vi "init.vi"(8 "error in":errorcluster, 10 "TBM module configuration in":refnum<class "TBM module configuration.lvclass">, 11 "Increment runtime in":refnum<class "Increment runtime.lvclass">) -> (0 "error out":errorcluster, 1 "data allocations":T1, 2 "execution settings":T4, 3 "Increment runtime out":refnum<class "Increment runtime.lvclass">)   [LabVIEW 2015, in "Increment runtime.lvclass"]
doc: "Provides an interface for initializing a module at runtime. While this interface performs no operations, a child should provide an override which may open any necessary references or sessions, allocate necessary memory, and perform any final configuration validataion before providing the full configuration <b>execution data</b> to the calling process."
uses:
  Increment runtime.lvclass
  <vilib>/NI/Tag Bus Module Framework/module configuration/TBM module configuration.lvclass
  <vilib>/NI/Tag Bus Module Framework/runtime/execution settings.ctl
  <vilib>/NI/Tag Bus Module Framework/channel/data tables.ctl
  <vilib>/NI/Tag Bus/dictionary/data dictionary.lvclass
  <vilib>/NI/Tag Bus/dictionary table pair.ctl
  <vilib>/NI/Tag Bus/table/data table.ctl
  configuration/Increment configuration.lvclass
  configuration/Increment configuration.lvclass/Increment configuration.ctl
  Runtime_Mapping.ctl
  <vilib>/NI/Tag Bus/tag/tag descriptor.lvclass/tag descriptor.ctl
  Increment runtime.lvclass/Increment runtime.ctl
  configuration/Read Lines.vi
  <vilib>/NI/Tag Bus/tag/read tag name.vi
  <vilib>/NI/Tag Bus/tag/read data type.vi
  <vilib>/NI/Tag Bus/dictionary/locate tag.vi
  <vilib>/NI/Tag Bus Module Framework/channel/TBM channel.lvclass
  <vilib>/NI/Tag Bus Module Framework/runtime/TBM module execution interface.lvclass
  <vilib>/NI/Tag Bus/tag bus.lvlib
  <vilib>/NI/Tag Bus/table/data table.lvlib
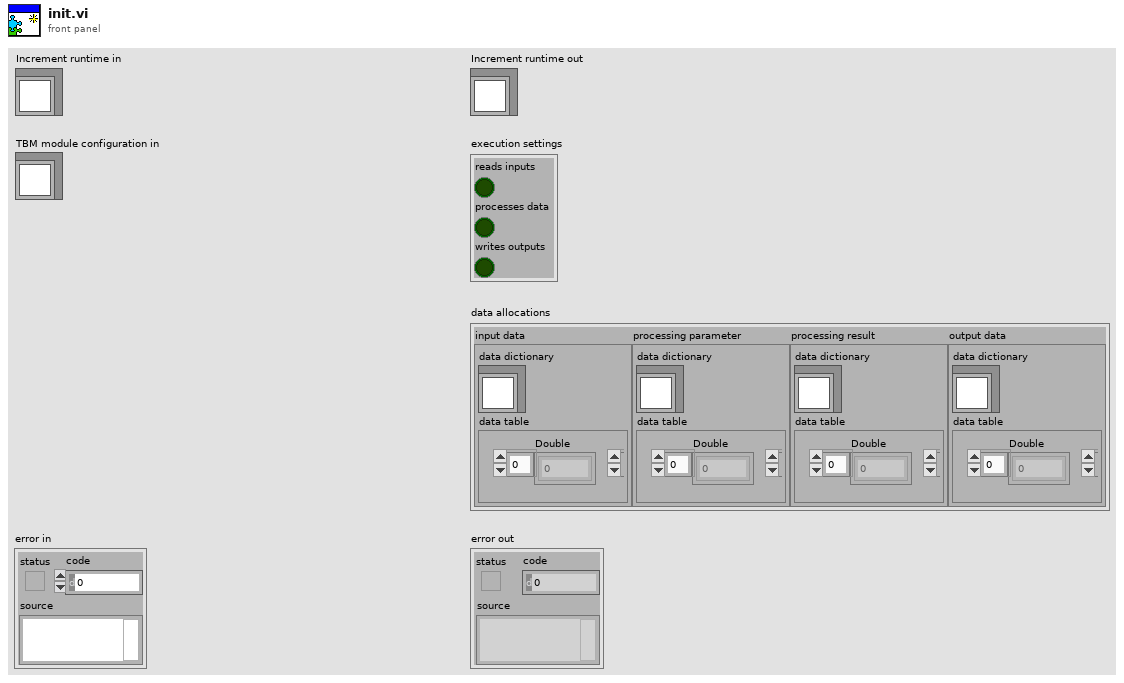
[diagram p1: front panel]
types:
  T1 = typedef "TBM channel.lvclass/data tables.ctl" = cluster{"input data":T2, "processing parameter":T2, "processing result":T2, "output data":T2}
  T2 = typedef "tag bus.lvlib/dictionary table pair.ctl" = cluster{"data dictionary":refnum<class "data dictionary.lvclass">, "data table":T3}
  T3 = typedef "tag bus.lvlib/data table.lvlib/data table.ctl" = cluster{"Double":dbl[], "Single":sgl[], "I64":i64[], "I32":i32[], "I16":i16[], "I8":i8[], "U64":u64[], "U32":u32[], "U16":u16[], "U8":u8[], "Boolean":bool[], "String":string[], "Array of Double":cluster{"DBL Array":dbl[]}[], "Array of Single":cluster{"SGL Array":sgl[]}[], "Array of I64":cluster{"I64 Array":i64[]}[], "Array of I32":cluster{"I32 Array":i32[]}[], "Array of I16":cluster{"I16 Array":i16[]}[], "Array of I8":cluster{"I8 Array":i8[]}[], "Array of U64":cluster{"U64 Array":u64[]}[], "Array of U32":cluster{"U32 Array":u32[]}[], "Array of U16":cluster{"U16 Array":u16[]}[], "Array of U8":cluster{"U8 Array":u8[]}[], "Array of Boolean":cluster{"Boolean Array":bool[]}[], "Array of String":cluster{"String Array":string[]}[]}
  T4 = typedef "TBM module execution interface.lvclass/execution settings.ctl" = cluster{"reads inputs":bool, "processes data":bool, "writes outputs":bool}
  T5 = typedef "Increment runtime.lvclass/Runtime_Mapping.ctl" = cluster{"In Index":i32, "Out Index":i32}
  T6 = typedef "Increment configuration.lvclass/Line.ctl" = cluster{"Name":string, "channel in":refnum<class "TBM channel.lvclass">, "channel out":refnum<class "TBM channel.lvclass">}
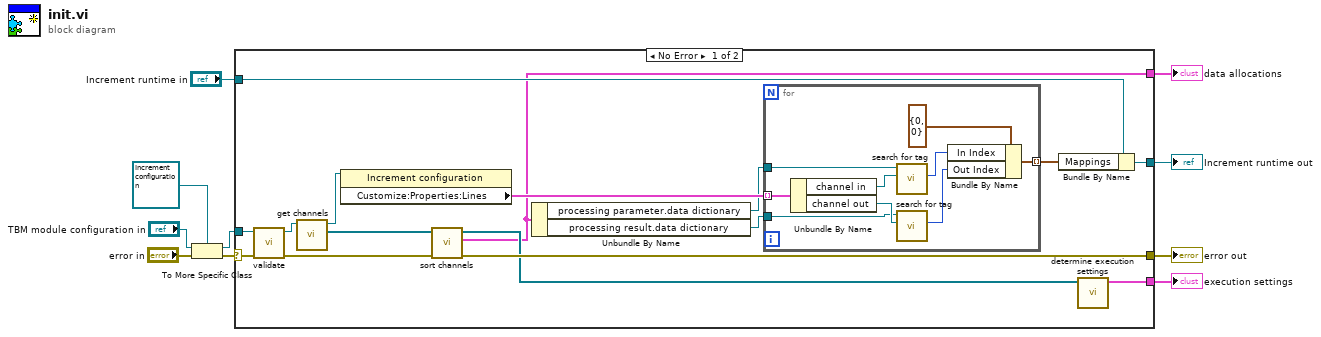
[diagram p0: block diagram]
diagram:
  n1 = To More Specific Class(target class=refnum<class "Increment configuration.lvclass"> refnum ("Synchronous module configuration"), reference="TBM module configuration in", error in="error in") -> (specific class reference=w9:refnum<class "Increment configuration.lvclass">, error out=w10:errorcluster)
  n2 = case shown="No Error" w10 {
    selector: w10 -> [w22 w36]
    tunnel: w9 -> [w21 _]
    tunnel: "Increment runtime in" -> [w17 w37]
    tunnel: [w16 w37] -> w4
    tunnel: [w26 w36] -> w3
    tunnel: [w14 _] -> w1
    tunnel: [w25 _] -> w2
    frame No Error {
      n3 = call-dynamic "validate.vi"("error in"=w22, "Increment configuration in"=w21) -> ("error out"=w23:errorcluster, "Increment configuration out"=w20:refnum<class "Increment configuration.lvclass">)  [unwired: 8 in]
      n4 = call-dynamic "get channels.vi"("Increment configuration in"=w20) -> ("channels"=w19:refnum<class "TBM channel.lvclass">[], "Increment configuration out"=w18:refnum<class "Increment configuration.lvclass">)  [unwired: 9 in]
      n5 = property class="Increment configuration"(reference=w18) -> ("Customize:Properties:Lines"=w15:T6[])  [unwired: 1 in, 2 out]
      n6 = call <vilib>:"sort channels.vi"("error in"=w23, "channels in"=w19) -> ("error out"=w26:errorcluster, "data allocations"=w14:T1, "channels out"=w24:refnum<class "TBM channel.lvclass">[])  [unwired: 7 in]
      n7 = Unbundle By Name(w14) -> ("processing parameter.data dictionary"=w13:refnum<class "data dictionary.lvclass">, "processing result.data dictionary"=w12:refnum<class "data dictionary.lvclass">)
      n8 = for {
        tunnel: w15 -> [w35] mode=indexing
        tunnel: w13 -> [w33]
        tunnel: w12 -> [w31]
        tunnel: [w30] -> w11 mode=indexing
        n9 = Unbundle By Name(w35) -> ("channel in"=w34:refnum<class "TBM channel.lvclass">, "channel out"=w32:refnum<class "TBM channel.lvclass">)
        n10 = call <vilib>:"search for tag.vi"("system tag"=w34, "data dictionary in"=w33) -> ("index"=w29:i32)  [unwired: 7 in, 2 out]
        n11 = call <vilib>:"search for tag.vi"("system tag"=w32, "data dictionary in"=w31) -> ("index"=w28:i32)  [unwired: 7 in, 2 out]
        n12 = Bundle By Name(cluster=T5 {"In Index"=0, "Out Index"=0} ("Mapping"), "In Index"=w29, "Out Index"=w28) -> (w30:T5)
      }
      n13 = Bundle By Name(cluster=w17, "Mappings"=w11) -> (w16:refnum<class "Increment runtime.lvclass">)
      n14 = call <vilib>:"determine execution settings.vi"("channels"=w24) -> ("execution settings"=w25:T4)  [unwired: 10 in]
    }
    frame Error {
    }
  }
  "error out" <- w3
  "Increment runtime out" <- w4
  "execution settings" <- w2
  "data allocations" <- w1
